vi "游泳.vi"(8 "error in (no error)":errorcluster caption="错误输入（无错误）", 11 "鸭子 输入":refnum<class "鸭子.lvclass">) -> (0 "error out":errorcluster caption="错误输出", 3 "鸭子 输出":refnum<class "鸭子.lvclass">)   [LabVIEW 2018, in "鸭子库.lvlib" / "鸭子.lvclass"]
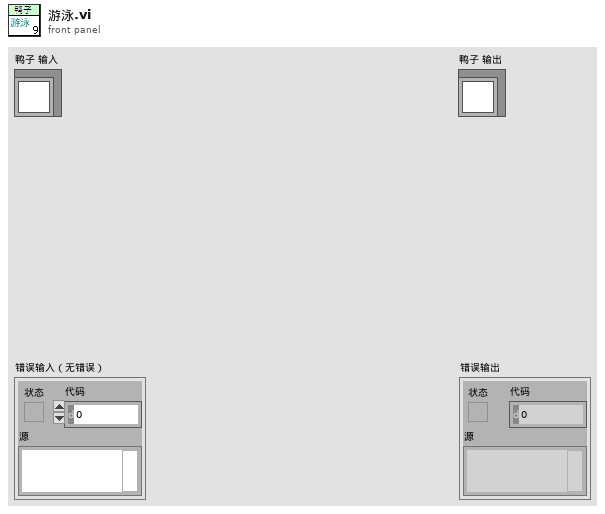
[diagram p1: front panel]
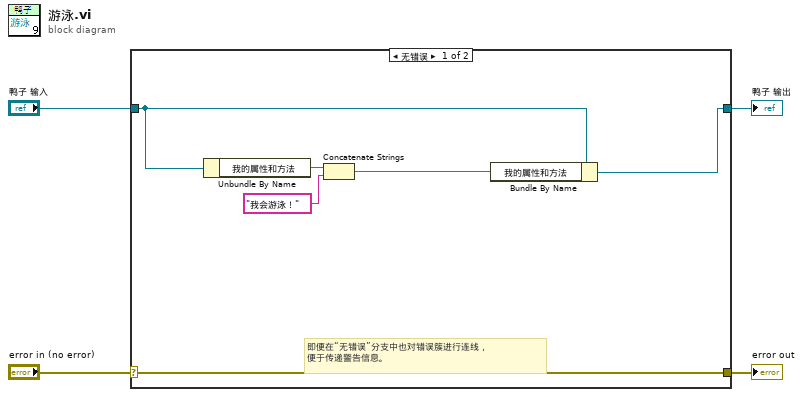
[diagram p0: block diagram]
diagram:
  n1 = case shown="无错误" "error in (no error)" {
    selector: "error in (no error)" -> [w10 w12]
    tunnel: [w10 w12] -> w3
    tunnel: [w6 w11] -> w1
    tunnel: "鸭子 输入" -> [w7 w11]
    frame No Error {
      # "即便在“无错误”分支中也对错误簇进行连线，\n便于传递警告信息。"
      n2 = Unbundle By Name(w7) -> ("我的属性和方法"=w9:string)
      n3 = Concatenate Strings(w9, "我会游泳！" ("字符串")) -> (w5:string)
      n4 = Bundle By Name(cluster=w7, "我的属性和方法"=w5) -> (w6:refnum<class "鸭子.lvclass">)
    }
    frame Error {
    }
  }
  "error out" <- w3
  "鸭子 输出" <- w1
